vi "Curtin1_FileListing.vi"(11 "Folder Path":path) -> (3 "Array":cluster{"Folder Path":path, "tags":string[]}[](array[cluster]))   [LabVIEW 2022 SP3]
uses:
  <vilib>/Utility/file.llb/Read Delimited Spreadsheet (string).vi
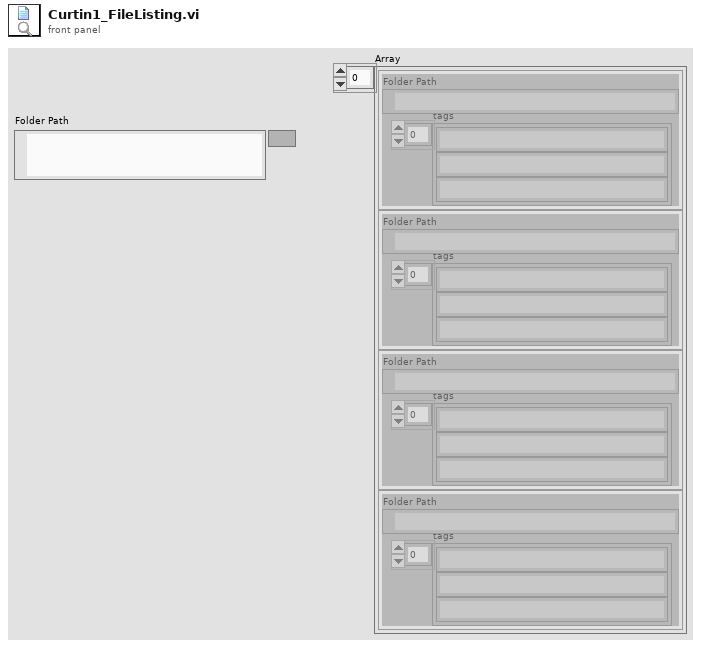
[diagram p1: front panel]
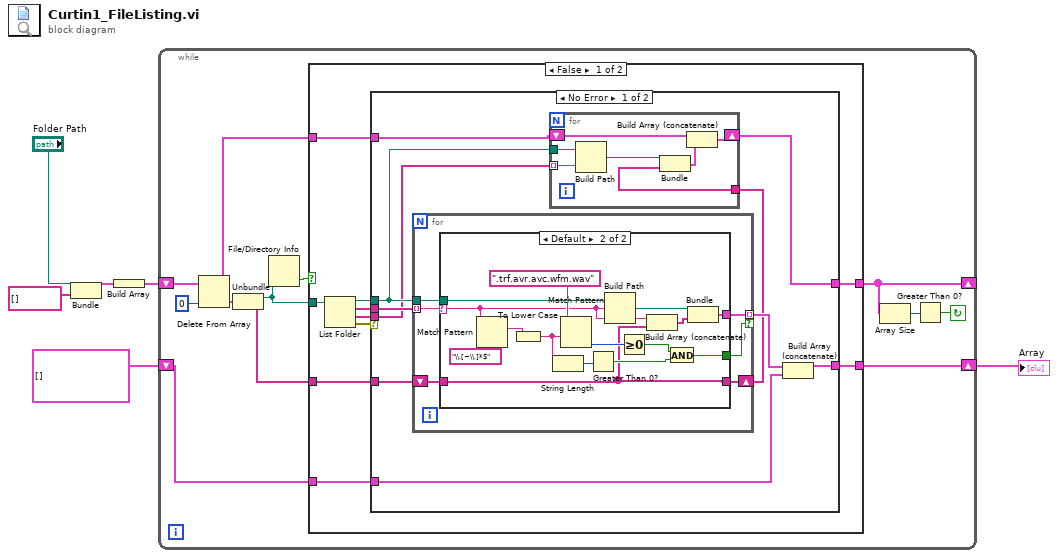
[diagram p0: block diagram]
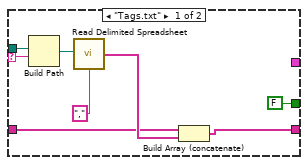
[diagram p2: hidden frame]
diagram:
  n1 = Bundle("Folder Path"="Folder Path", string[] []) -> (w3:cluster{"Folder Path":path, string[]})  [unwired: 1 in]
  n2 = Build Array(w3) -> (w6:cluster{"Folder Path":path, string[]}[])
  n3 = while {
    shift-right: [w12] -> _
    shift-left: w6 -> [w18]
    shift-right: [w11] -> w2
    shift-left: cluster{"appended path":path, string[]}[] [] -> [w9]
    stop <- w13 continue-if-true
    n4 = Delete From Array(array=w18, index=0) -> (deleted portion=w8:cluster{"Folder Path":path, string[]}, array with subset deleted=w10:cluster{"Folder Path":path, string[]}[])  [unwired: 1 in]
    n5 = Unbundle(w8) -> ("Folder Path"=w15:path, w7:string[])
    n6 = File/Directory Info(path=w15) -> (shortcut=w17:bool)  [unwired: 1 in, 6 out]
    n7 = case shown="False" w17 {
      tunnel: w15 -> [w28 _]
      tunnel: w10 -> [w24 w78]
      tunnel: [w23 w78] -> w12
      tunnel: [w21 w77] -> w11
      tunnel: w9 -> [w20 w77]
      tunnel: w7 -> [w19 _]
      frame False {
        n8 = List Folder(path=w28) -> (path out=w25:path, filenames=w26:string[], folder names=w22:string[], error out=w27:errorcluster)  [unwired: 3 in]
        n9 = case shown="No Error" w27 {
          tunnel: w26 -> [w37 _]
          tunnel: w25 -> [w38 _]
          tunnel: w24 -> [w36 w76]
          tunnel: [w34 w76] -> w23
          tunnel: w22 -> [w35 _]
          tunnel: [w31 w75] -> w21
          tunnel: w20 -> [w33 w75]
          tunnel: w19 -> [w30 _]
          frame No Error {
            n10 = for {
              tunnel: w37 -> [w48] mode=indexing
              tunnel: w38 -> [w51]
              tunnel: [w50] -> w32 mode=indexing if=w49
              shift-right: [w46] -> w29
              shift-left: w30 -> [w47]
              n11 = case shown="Default" w48 {
                selector: w48 -> [w57 w61]
                tunnel: w51 -> [w58 w74]
                tunnel: [_ w70] -> w50
                tunnel: [FALSE w65] -> w49
                tunnel: w47 -> [w53 w60]
                tunnel: [w52 w60] -> w46
                frame "Tags.txt" {
                  n12 = Build Path(base path=w58, name or relative path=w57) -> (appended path=w56:path)
                  n13 = call-poly <vilib>:"Read Delimited Spreadsheet.vi"("file path (dialog if empty)"=w56, "delimiter (\\t)"="," ("delimiter (\\t)")) -> ("first row"=w55:string[])  [unwired: 8 in, 5 out]
                  n14 = Build Array (concatenate)(w53, w55) -> (w52:string[])
                }
                frame Default {
                  n15 = Match Pattern(string=w61, regular expression="\\.[~\\.]*$") -> (match substring=w62:string)  [unwired: 4 out]
                  n16 = To Lower Case(string=w62) -> (all lower case string=w63:string)
                  n17 = String Length(string=w63) -> (length=w64:i32)
                  n18 = Match Pattern(string=".trf.avr.avc.wfm.wav" ("regular expression"), regular expression=w63) -> (offset past match=w69:i32)  [unwired: 1 in, 3 out]
                  n19 = Greater Than 0?(x=w64) -> (x > 0?=w67:bool)
                  n20 = Build Path(base path=w74, name or relative path=w61) -> (appended path=w71:path)
                  n21 = Greater Or Equal To 0?(x=w69) -> (x >= 0?=w66:bool)
                  n22 = Build Array (concatenate)(w61, w60) -> (w68:string[])
                  n23 = And(x=w66, y=w67) -> (x .and. y?=w65:bool)
                  n24 = Bundle("appended path"=w71, w68) -> (w70:cluster{"appended path":path, string[]})  [unwired: 1 in]
                }
              }
            }
            n25 = for {
              tunnel: w38 -> [w45]
              tunnel: w35 -> [w44] mode=indexing
              shift-right: [w40] -> w34
              shift-left: w36 -> [w42]
              tunnel: w29 -> [w39]
              n26 = Build Path(base path=w45, name or relative path=w44) -> (appended path=w43:path)
              n27 = Bundle("appended path"=w43, w39) -> (w41:cluster{"appended path":path, string[]})  [unwired: 1 in]
              n28 = Build Array (concatenate)(w42, w41) -> (w40:cluster{"appended path":path, string[]}[])
            }
            n29 = Build Array (concatenate)(w32, w33) -> (w31:cluster{"appended path":path, string[]}[])
          }
          frame Error {
          }
        }
      }
      frame True {
      }
    }
    n30 = Array Size(array=w12) -> (size(s)=w14:i32)
    n31 = Greater Than 0?(x=w14) -> (x > 0?=w13:bool)
  }
  "Array" <- w2
